vi "Untitled 23.vi"() -> ()   [LabVIEW 2019]
uses:
  Generated_client/RPC Messages/routeguide_Rectangle.ctl
  Generated_client/RPC Messages/routeguide_Point.ctl
  <vilib>/gRPC/LabVIEW gRPC Library/Shared/Any.ctl
  Generated_client/RPC Messages/routeguide_Feature.ctl
  Generated_client/Generated_client.lvlib
  <vilib>/gRPC/LabVIEW gRPC Library/grpc-lvsupport-release.lvlib
panel:
  out "Array":T1[](array[typedef])
  out "error out":errorcluster
  out "errorDetails":T3
  out "Success":bool
  in  "Request Data":T4
  in  "address":string
  in  "error in":errorcluster
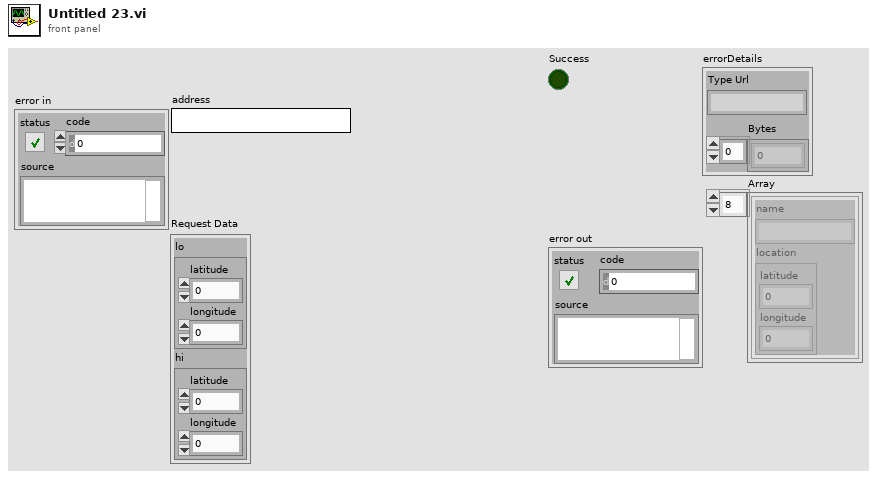
[diagram p1: front panel]
types:
  T1 = typedef "Generated_client.lvlib/routeguide_Feature.ctl" = cluster{"name":string, "location":T2}
  T2 = typedef "Generated_client.lvlib/routeguide_Point.ctl" = cluster{"latitude":i32, "longitude":i32}
  T3 = typedef "grpc-lvsupport-release.lvlib/Any.ctl" = cluster{"Type Url":string, "Bytes":u8[]}
  T4 = typedef "Generated_client.lvlib/routeguide_Rectangle.ctl" = cluster{"lo":T2, "hi":T2}
  T5 = typedef "grpc-lvsupport-release.lvlib/grpcId.ctl" = u64
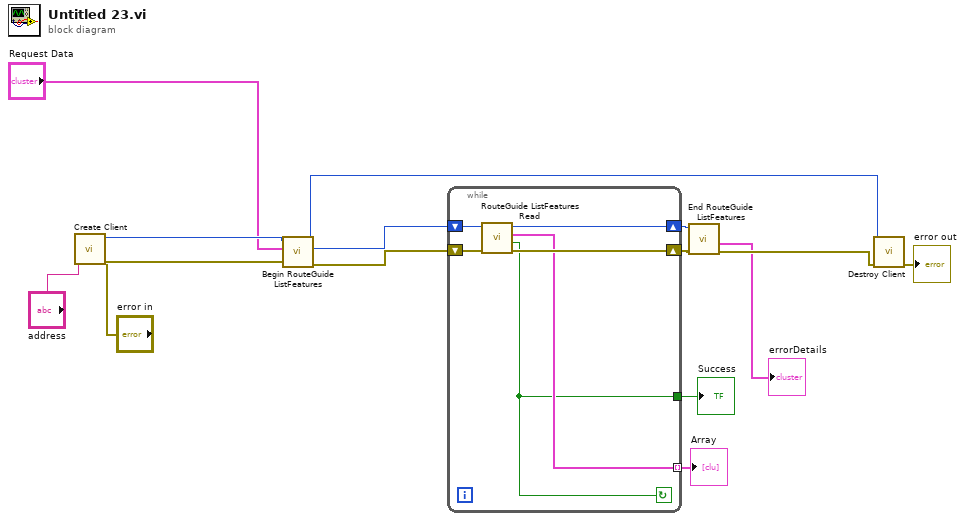
[diagram p0: block diagram]
diagram:
  n1 = call "Create Client.vi"("error in"="error in", "address"="address") -> ("error out"=w11:errorcluster, "gRPC ID Out"=w15:T5)  [unwired: 8 in]
  n2 = call "Begin RouteGuide ListFeatures.vi"("error in"=w11, "Request Data"="Request Data", "gRPC ID"=w15) -> ("error out"=w10:errorcluster, "Call Id Out"=w14:T5, "gRPC ID out"=w12:T5)  [unwired: 6 in]
  n3 = while {
    shift-right: [w20] -> w13
    shift-left: w14 -> [w21]
    shift-right: [w18] -> w9
    shift-left: w10 -> [w19]
    tunnel: [w17] -> w1 mode=indexing
    tunnel: [w16] -> w2
    stop <- w16 continue-if-true
    n4 = call "RouteGuide ListFeatures Read.vi"("error in"=w19, "Call ID in"=w21) -> ("error out"=w18:errorcluster, "Success"=w16:bool, "Response Data"=w17:T1, "Call ID"=w20:T5)  [unwired: 6 in]
  }
  "Success" <- w2
  "Array" <- w1
  n5 = call "End RouteGuide ListFeatures.vi"("error in"=w9, "Call ID in"=w13) -> ("error out"=w8:errorcluster, "errorDetails"=→"errorDetails":T3)  [unwired: 8 in]
  n6 = call "Destroy Client.vi"("error in"=w8, "gRPC ID"=w12) -> ("error out"=→"error out":errorcluster)  [unwired: 9 in]
